vi "Angle From Origin.vi"(10 "Y":dbl, 11 "X":dbl) -> (2 "Above Y Axis?":bool, 3 "Angle":dbl)   [LabVIEW 2013]
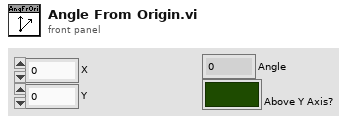
[diagram p1: front panel]
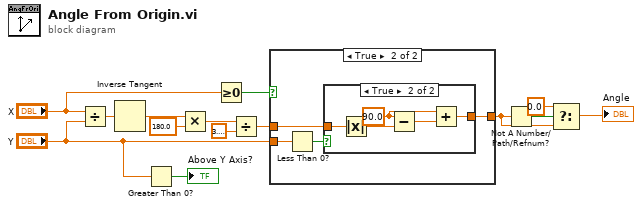
[diagram p0: block diagram]
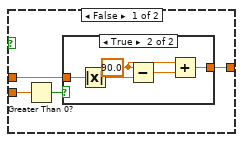
[diagram p2: hidden frame]
diagram:
  n1 = Divide(x="X", y="Y") -> (x/y=w13:dbl)
  n2 = Inverse Tangent(1:w13) -> (0:w11:dbl)
  n3 = Greater Than 0?(x="Y") -> (x > 0?=→"Above Y Axis?":bool)
  n4 = Multiply(x=w11, y=180.0) -> (x*y=w9:dbl)
  n5 = Greater Or Equal To 0?(x="X") -> (x >= 0?=w10:bool)
  n6 = Divide(x=w9, y=3.141592653589793) -> (x/y=w8:dbl)
  n7 = case shown="True" w10 {
    tunnel: "Y" -> [w16 w28]
    tunnel: w8 -> [w17 w26]
    tunnel: [w15 w25] -> w4
    frame False {
      n8 = Greater Than 0?(x=w16) -> (x > 0?=w18:bool)
      n9 = case shown="True" w18 {
        tunnel: w17 -> [w19 w24]
        tunnel: [w19 w20] -> w15
        frame False {
        }
        frame True {
          w21 = 90.0 ("x")
          n10 = Absolute Value(x=w24) -> (abs(x)=w23:dbl)
          n11 = Subtract(x=w21, y=w23) -> (x-y=w22:dbl)
          n12 = Add(x=w21, y=w22) -> (x+y=w20:dbl)
        }
      }
    }
    frame True {
      n13 = Less Than 0?(x=w28) -> (x < 0?=w27:bool)
      n14 = case shown="True" w27 {
        tunnel: w26 -> [w29 w34]
        tunnel: [w29 w30] -> w25
        frame False {
        }
        frame True {
          w31 = 90.0 ("x")
          n15 = Absolute Value(x=w34) -> (abs(x)=w33:dbl)
          n16 = Subtract(x=w31, y=w33) -> (x-y=w32:dbl)
          n17 = Add(x=w31, y=w32) -> (x+y=w30:dbl)
        }
      }
    }
  }
  n18 = Not A Number/Path/Refnum?(number/path/refnum=w4) -> (NaN/Path/Refnum?=w6:bool)
  n19 = Select(t=0.0, s=w6, f=w4) -> (s? t:f=→"Angle":dbl)
